vi "Maths - Round to X Decimal Places.vi"(0 "Floating In":dbl format="%#_10g", 1 "Decimal Places (2)":i32=2) -> (2 "Floating Out":dbl format="%#_10g")   [LabVIEW 2010]
doc: "Rounds a floating point number to a defined number of decimal places."
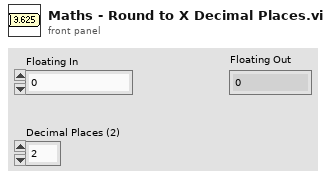
[diagram p1: front panel]
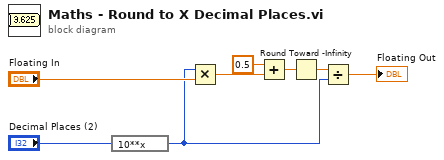
[diagram p0: block diagram]
diagram:
  n1 = expression code="10**x"("Decimal Places (2)") -> (w3:i32)
  n2 = Multiply(x=w3, y="Floating In") -> (x*y=w6:dbl)
  n3 = Add(x=0.5, y=w6) -> (x+y=w4:dbl)
  n4 = Round Toward -Infinity(1:w4) -> (0:w1:dbl)
  n5 = Divide(x=w1, y=w3) -> (x/y=→"Floating Out":dbl)
